vi "PDLM_CloseDevice.vi"(8 "error in (no error)":errorcluster, 11 "USBIdx":i32) -> (0 "error out":errorcluster, 3 "return type":i32)   [LabVIEW 2019]
uses:
  <userlib>/TaikoLaser/PDLM_DllPath_global.vi
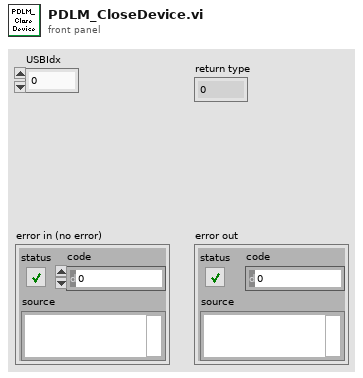
[diagram p1: front panel]
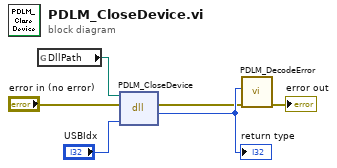
[diagram p0: block diagram]
diagram:
  n1 = global read "PDLM_DllPath_global.vi" "DllPath"() -> (w2:path)
  n2 = dll-call lib="M:/_dev/progs/LabVIEW/_lib/PQ/Taiko/pdlm_lib.dll" fn="PDLM_CloseDevice"(path in=w2, error in="error in (no error)", "USBIdx"="USBIdx") -> (error out=w4:errorcluster, "return type"=w5:i32)  [unwired: 2 in, 1 out]
  "return type" <- w5
  n3 = call <userlib>:"PDLM_DecodeError.vi"("error in (no error)"=w4, "code"=w5) -> ("error out"=→"error out":errorcluster)  [unwired: 7 in, 2 out]
